vi "SetExposure.vi"(7 "error in (no error)":errorcluster, 9 "Exposure[ms]":dbl format="%#_13g", 10 "Handle in":u32) -> (0 "error out":errorcluster, 1 "framerate":dbl, 2 "exposure":dbl, 3 "Handle out":u32)   [LabVIEW 2015]
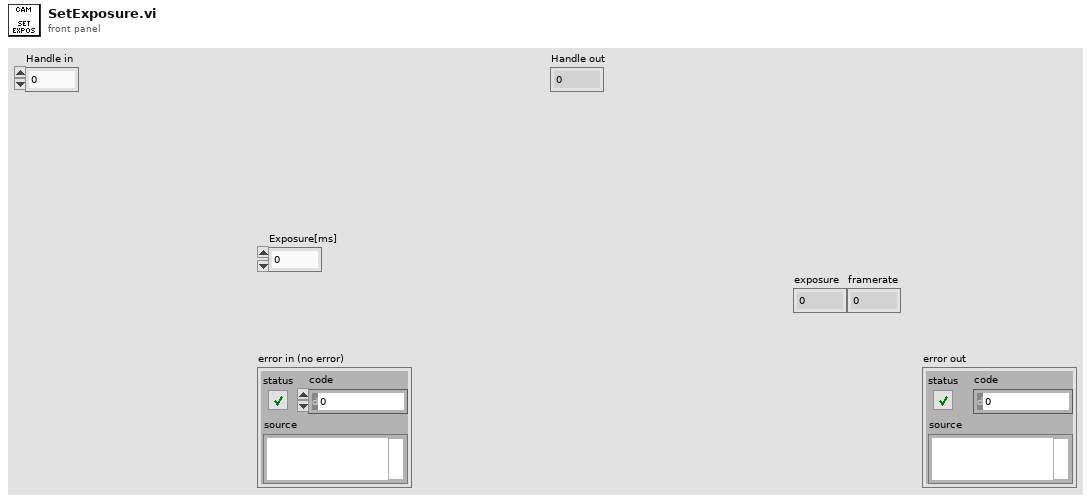
[diagram p1: front panel]
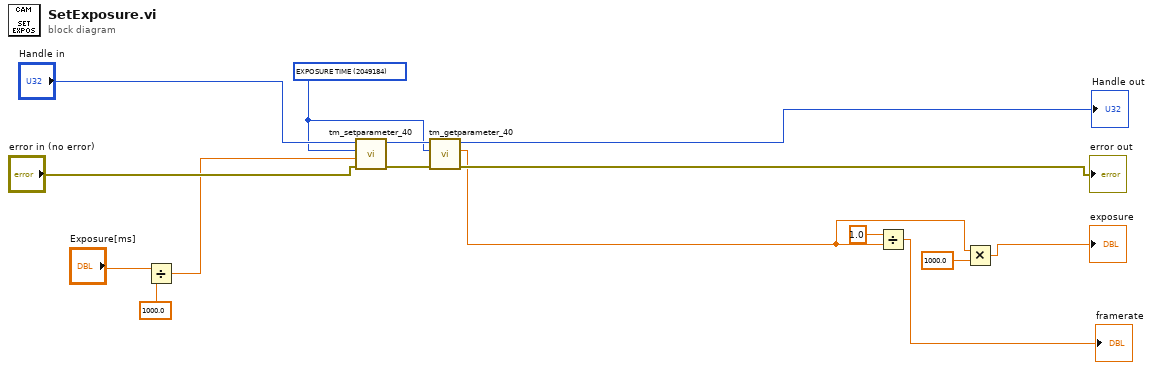
[diagram p0: block diagram]
diagram:
  w11 = u32 2049184 items=["SENSOR MODE"=4212128, "READOUT SPEED"=4211872, "READOUT DIRECTION"=4211904, "TRIGGER GLOBAL EXPOSURE"=2049680, "TRIGGER DELAY"=1066480, "INTERNAL TRIGGER HANDLING"=1066496, "SYNC READOUT SYSTEM BLANK"=1066528, "SENSOR TEMPERATURE"=2115232, "SENSOR COOLER STATUS"=2115280, "EXPOSURE TIME"=2049184, "DEFECT CORRECT MODE"=4670368, "BINNING"=4215968, "INTERNAL LINE SPEED"=4226000, "INTERNAL LINE INTERVAL"=4226016, "NUMBER OF OUTPUT TRIGGER CONNECTOR"=1852320, "OUTPUT TRIGGER SOURCE[0]"=1852576, "OUTPUT TRIGGER SOURCE[1]"=1852832, "OUTPUT TRIGGER SOURCE[2]"=1853088, "OUTPUT TRIGGER POLARITY[0]"=1852592, "OUTPUT TRIGGER POLARITY[1]"=1852848, "OUTPUT TRIGGER POLARITY[2]"=1853104, "OUTPUT TRIGGER ACTIVE[0]"=1852608, "OUTPUT TRIGGER ACTIVE[1]"=1852864, "OUTPUT TRIGGER ACTIVE[2]"=1853120, "OUTPUT TRIGGER DELAY[0]"=1852624, "OUTPUT TRIGGER DELAY[1]"=1852880, "OUTPUT TRIGGER DELAY[2]"=1853136, "OUTPUT TRIGGER PERIOD[0]"=1852640, "OUTPUT TRIGGER PERIOD[1]"=1852896, "OUTPUT TRIGGER PERIOD[2]"=1853152, "OUTPUT TRIGGER KIND[0]"=1852656, "OUTPUT TRIGGER KIND[1]"=1852912, "OUTPUT TRIGGER KIND[2]"=1853168, "OUTPUT TRIGGER BASE SENSOR[0]"=1852672, "OUTPUT TRIGGER BASE SENSOR[1]"=1852928, "OUTPUT TRIGGER BASE SENSOR[2]"=1853184, "OUTPUT TRIGGER PRE HSYNC COUNT"=1852704] ("Parameter")
  n1 = Divide(x="Exposure[ms]", y=1000.0) -> (x/y=w4:dbl)
  n2 = call <userlib>:"tm_setparameter_40.vi"("error in (no error)"="error in (no error)", "Value in"=w4, "Parameter"=w11, "Handle in"="Handle in") -> ("error out"=w13:errorcluster, "Handle out"=w12:u32)  [unwired: 6 in]
  n3 = call <userlib>:"tm_getparameter_40.vi"("error in (no error)"=w13, "Parameter"=w11, "Handle in"=w12) -> ("error out"=→"error out":errorcluster, "Value out"=w3:dbl, "Handle out"=→"Handle out":u32)  [unwired: 6 in]
  n4 = Divide(x=1.0, y=w3) -> (x/y=→"framerate":dbl)
  n5 = Multiply(x=w3, y=1000.0) -> (x*y=→"exposure":dbl)
